vi "CreateSlotNode.vi"(7 "DOM Document":refnum<k20>, 8 "Error In":errorcluster, 11 "Slot Configuration":T1) -> (0 "Error Out":errorcluster, 3 "Bank Channel Node":refnum<k20>)   [LabVIEW 2012]
uses:
  SlotConfiguration.ctl
  BankConfiguration.ctl
  libs/LV-Utilities/LV-Utilities.lvlib
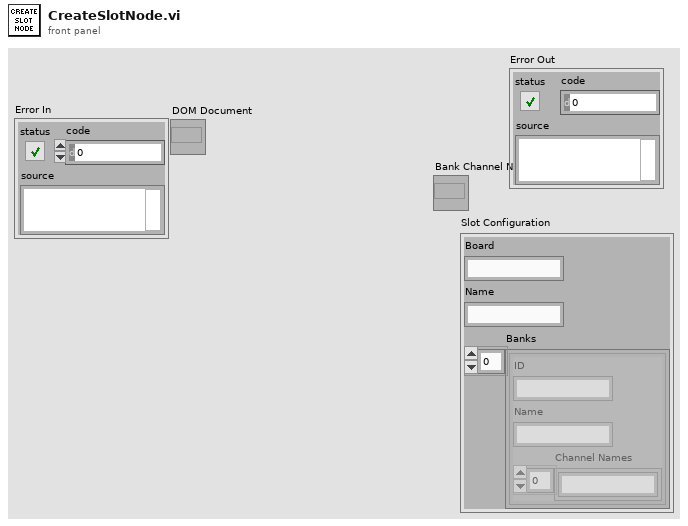
[diagram p1: front panel]
types:
  T1 = typedef "SlotConfiguration.ctl" = cluster{"Board":string, "Name":string, "Banks":T2[]}
  T2 = typedef "BankConfiguration.ctl" = cluster{"ID":string, "Name":string, "Channel Names":string[]}
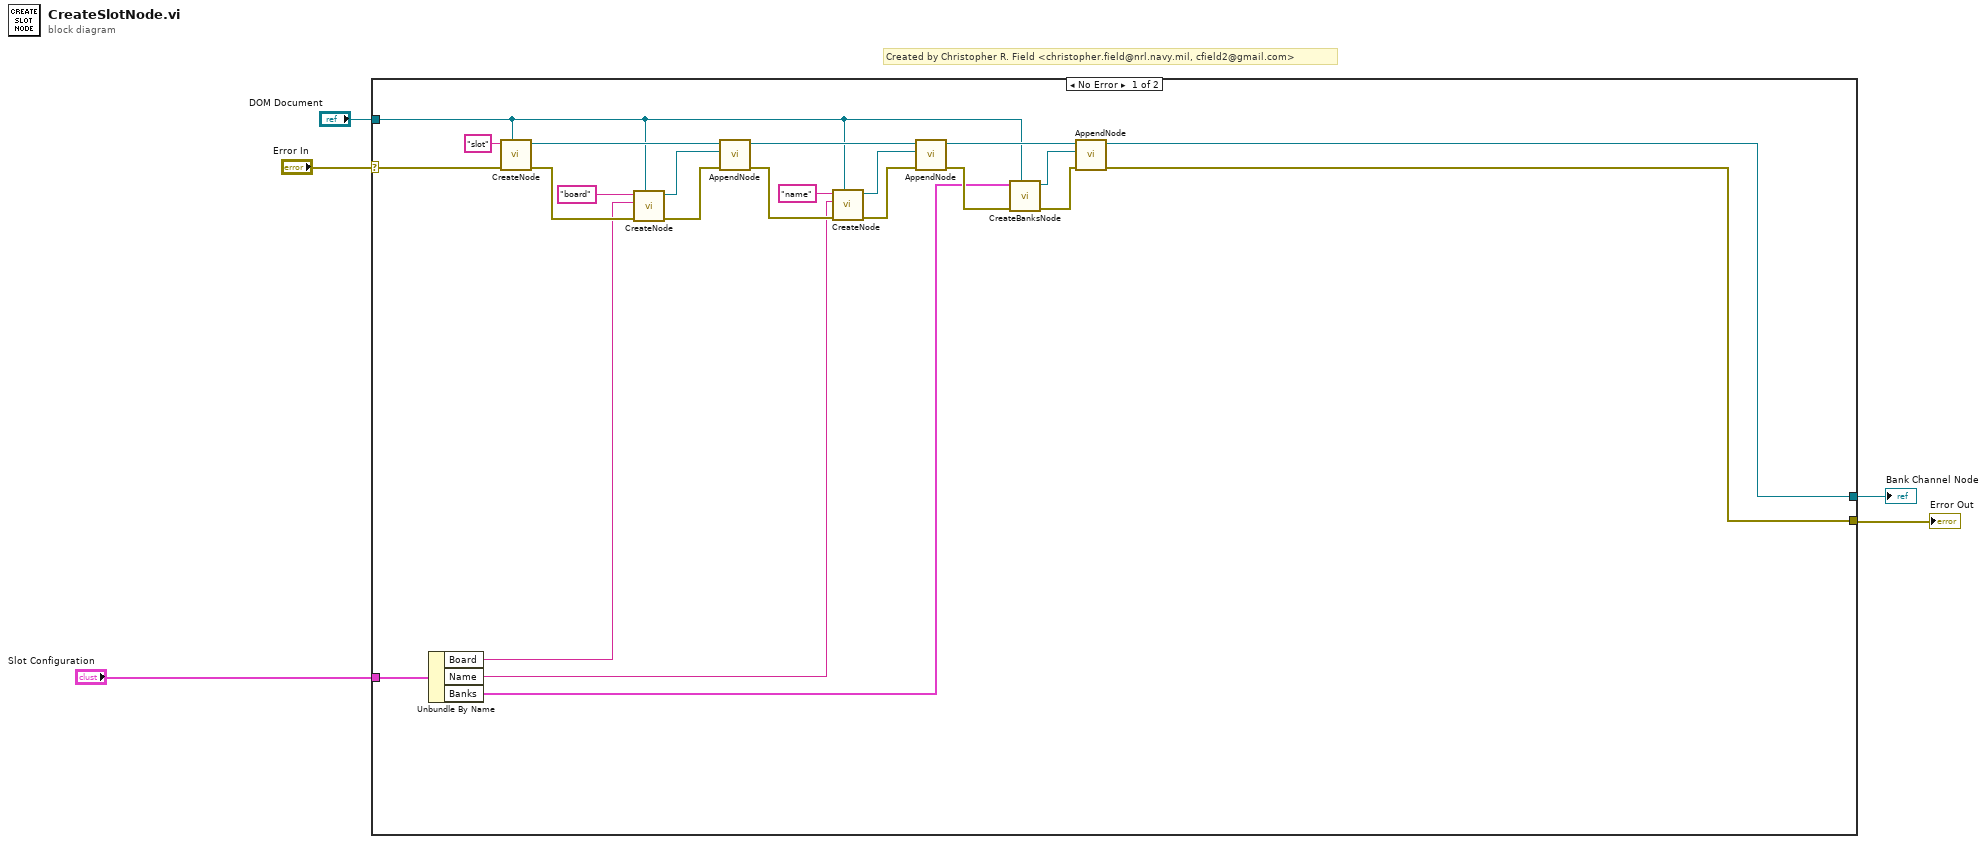
[diagram p0: block diagram]
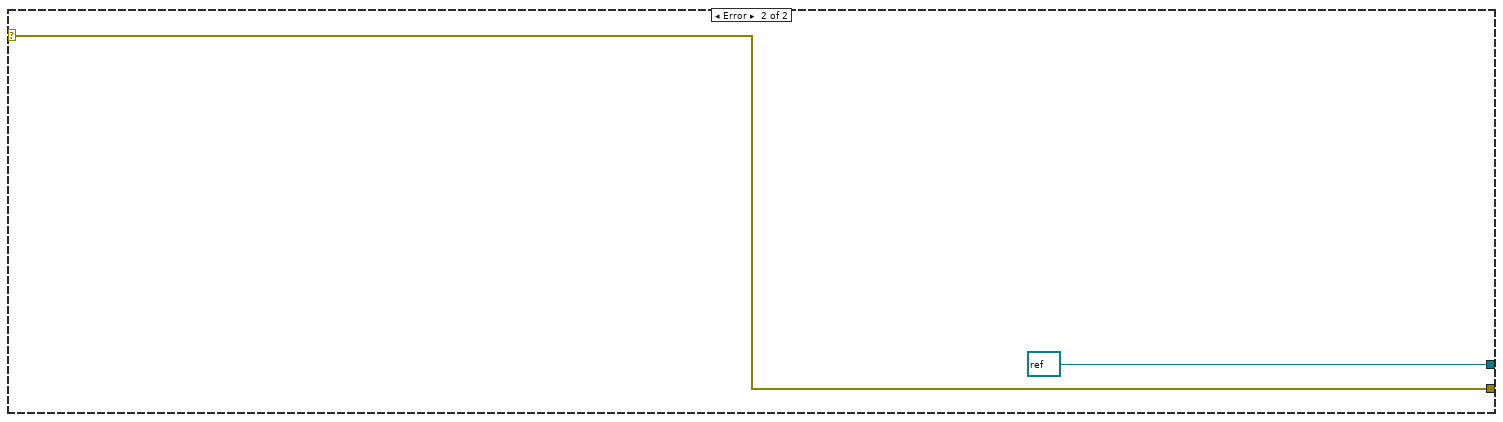
[diagram p2: hidden frame]
diagram:
  # "Created by Christopher R. Field <christopher.field@nrl.navy.mil, cfield2@gmail.com>"
  n1 = case shown="No Error" "Error In" {
    selector: "Error In" -> [w28 w30]
    tunnel: "DOM Document" -> [w9 _]
    tunnel: [w12 w30] -> w3
    tunnel: [w13 refnum<k20> refnum ("Wirings Node 2")] -> w2
    tunnel: "Slot Configuration" -> [w11 _]
    frame No Error {
      n2 = Unbundle By Name(w11) -> ("Board"=w24:string, "Name"=w18:string, "Banks"=w8:T2[])
      n3 = call "CreateNode.vi"("DOM Document"=w9, "Error In"=w28, "Tag Name"="slot") -> ("Error out"=w26:errorcluster, "Node"=w23:refnum<k20>)  [unwired: 7 in]
      n4 = call "CreateNode.vi"("DOM Document"=w9, "Error In"=w26, "Text"=w24, "Tag Name"="board") -> ("Error out"=w21:errorcluster, "Node"=w22:refnum<k20>)  [unwired: 6 in]
      n5 = call "AppendNode.vi"("Error In"=w21, "Child Node"=w22, "Parent Node In"=w23) -> ("Error Out"=w20:errorcluster, "Parent Node Out"=w17:refnum<k20>)  [unwired: 7 in]
      n6 = call "CreateNode.vi"("DOM Document"=w9, "Error In"=w20, "Text"=w18, "Tag Name"="name") -> ("Error out"=w15:errorcluster, "Node"=w16:refnum<k20>)  [unwired: 6 in]
      n7 = call "AppendNode.vi"("Error In"=w15, "Child Node"=w16, "Parent Node In"=w17) -> ("Error Out"=w10:errorcluster, "Parent Node Out"=w14:refnum<k20>)  [unwired: 7 in]
      n8 = call "CreateBanksNode.vi"("DOM Document"=w9, "Error In"=w10, "Banks"=w8) -> ("Error Out"=w6:errorcluster, "Banks Node"=w7:refnum<k20>)  [unwired: 7 in]
      n9 = call "AppendNode.vi"("Error In"=w6, "Child Node"=w7, "Parent Node In"=w14) -> ("Error Out"=w12:errorcluster, "Parent Node Out"=w13:refnum<k20>)  [unwired: 7 in]
    }
    frame Error {
    }
  }
  "Bank Channel Node" <- w2
  "Error Out" <- w3
